vi "Init.vi"(11 "Msg Type Strategy in":refnum<class "Msg Type Strategy.lvclass">) -> (0 "error out":errorcluster, 3 "Msg Type Strategy out":refnum<class "Msg Type Strategy.lvclass">)   [LabVIEW 2021, in "jettl.lvlib" / "Msg Type Strategy.lvlib" / "Msg Type Strategy.lvclass"]
uses:
  Msg Type Strategy.lvclass
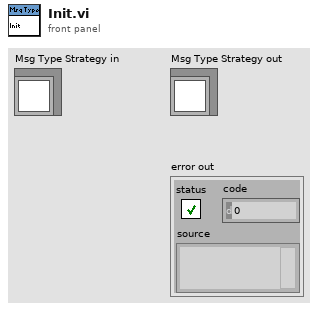
[diagram p1: front panel]
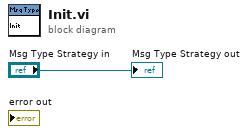
[diagram p0: block diagram]
diagram:
  "Msg Type Strategy out" <- "Msg Type Strategy in"
